vi "Find Plugins.vi"(11 "Plugin path":path=path "Plugin path") -> (2 "Plugin":string[](array[string]))   [LabVIEW 2025, in "HW Engine.lvlib" / "HW Engine.lvclass"]
uses:
  HW Engine.lvclass
  HW Engine.lvclass/HW Engine.ctl
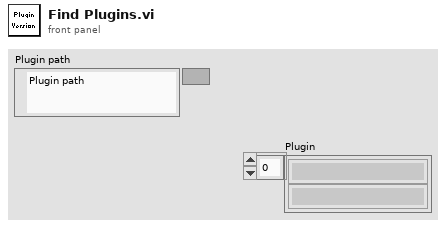
[diagram p1: front panel]
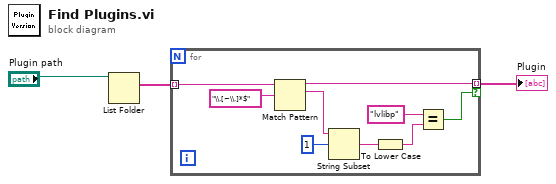
[diagram p0: block diagram]
diagram:
  n1 = List Folder(path="Plugin path") -> (filenames=w3:string[])  [unwired: 3 in, 3 out]
  n2 = for {
    tunnel: w3 -> [w4] mode=indexing
    tunnel: [w6] -> w2 mode=indexing if=w5
    n3 = Match Pattern(string=w4, regular expression="\\.[~\\.]*$") -> (before substring=w6:string, match substring=w11:string)  [unwired: 3 out]
    n4 = String Subset(string=w11, offset (0)=1) -> (substring=w9:string)  [unwired: 1 out]
    n5 = To Lower Case(string=w9) -> (all lower case string=w8:string)
    n6 = Equal?(x="lvlibp", y=w8) -> (x = y?=w5:bool)
  }
  "Plugin" <- w2
